vi "CSM - Sync Configuration Variables to File.vi"(4 "Write UnSupported Datatype?(F)":bool, 5 "All Temp Variable to Default Ini(F)":bool, 8 "error in (no error)":errorcluster) -> (2 "error out":errorcluster)   [LabVIEW 2017, in "INI-Static-Variable-Support.lvlib"]
uses:
  INI-Static-Variable-Support.lvlib
  _Support/_fgv-oper.ctl
  _Support/global-csm-ini-db-change-flag.vi
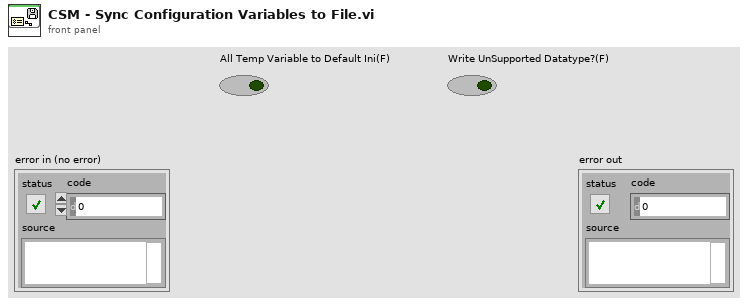
[diagram p1: front panel]
types:
  T1 = typedef "INI-Static-Variable-Support.lvlib/_fgv-oper.ctl" = enum16{"Read", "Write", "Sync", "Sessions", "List Keys", "Load", "List Files", "List Variables", "List Permanent Variables", "Mark Temp Variable as Permenent", "unload", "INIConfig(Memory)", "Reset", "Restore Variable Value"}
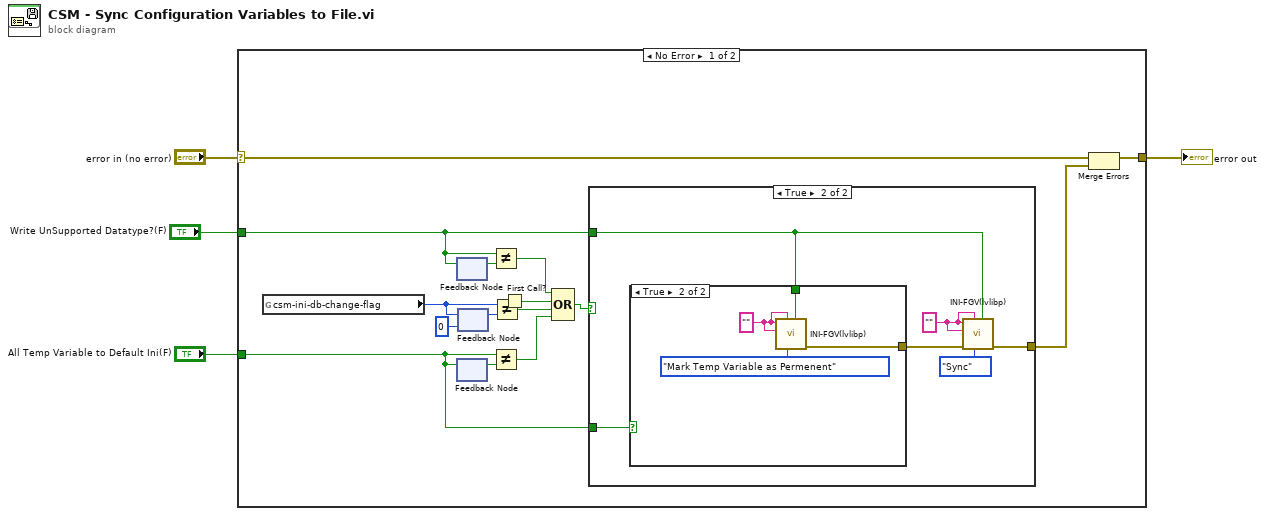
[diagram p0: block diagram]
diagram:
  n1 = case shown="No Error" "error in (no error)" {
    selector: "error in (no error)" -> [w18 w30]
    tunnel: [w19 w30] -> w4
    tunnel: "All Temp Variable to Default Ini(F)" -> [w8 _]
    tunnel: "Write UnSupported Datatype?(F)" -> [w6 _]
    frame No Error {
      n2 = global read "global-csm-ini-db-change-flag.vi" "csm-ini-db-change-flag"() -> (w17:u64)
      n3 = feedback #1() -> (w7:bool)  [unwired: 1 in]
      n4 = feedback-in #1(w6) -> ()
      n5 = feedback #2() -> (w10:bool)  [unwired: 1 in]
      n6 = feedback-in #2(w8) -> ()
      n7 = feedback #3(u64 0 ("csm-ini-db-change-flag")) -> (w16:u64)
      n8 = feedback-in #3(w17) -> ()
      n9 = Not Equal?(x=w6, y=w7) -> (x != y?=w5:bool)
      n10 = Not Equal?(x=w8, y=w10) -> (x != y?=w9:bool)
      n11 = Not Equal?(x=w17, y=w16) -> (x != y?=w15:bool)
      n12 = First Call?() -> (First Call?: T/F=w14:bool)
      n13 = Compound Arithmetic op=OR(w5, w14, w15, w9) -> (w13:bool)
      n14 = case shown="True" w13 {
        tunnel: [_ w24] -> w12
        tunnel: w8 -> [_ w22]
        tunnel: w6 -> [_ w21]
        frame False {
        }
        frame True {
          w20 = "" (">> Variable Name >>")
          n15 = case shown="True" w22 {
            tunnel: [_ w28] -> w23
            tunnel: w21 -> [_ w27]
            frame False {
            }
            frame True {
              w26 = "" (">> Variable Name >>")
              n16 = call "INI-FGV(lvlibp).vi"("Write If not found?"=w27, "Enum"=_fgv-oper."Mark Temp Variable as Permenent", "Prefered Section"=w26, ">> Default Value >>"=w26, ">> Variable Name >>"=w26) -> ("error out"=w28:errorcluster)  [unwired: 3 in, 3 out]
            }
          }
          n17 = call "INI-FGV(lvlibp).vi"("Write If not found?"=w21, "Enum"=_fgv-oper."Sync", "Prefered Section"=w20, "error IN"=w23, ">> Default Value >>"=w20, ">> Variable Name >>"=w20) -> ("error out"=w24:errorcluster)  [unwired: 2 in, 3 out]
        }
      }
      n18 = Merge Errors(w18, w12) -> (w19:errorcluster)
    }
    frame Error {
    }
  }
  "error out" <- w4
